vi "Wire Read Attributes.vi"(8 "error in (no error)":errorcluster, 9 "Controls":refnum<vi>[](array[refnum]), 10 "Cluster Refnum":refnum<vi>, 11 "VI in":refnum<vi>) -> (0 "error out":errorcluster, 3 "VI out":refnum<vi>)   [LabVIEW 2020, in "Message Maker.lvlib"]
uses:
  Message Maker.lvlib
  <vilib>/Utility/miscctls.llb/LVPositionTypeDef.ctl
  <vilib>/Utility/traverseref.llb/TRef TravTarget.ctl
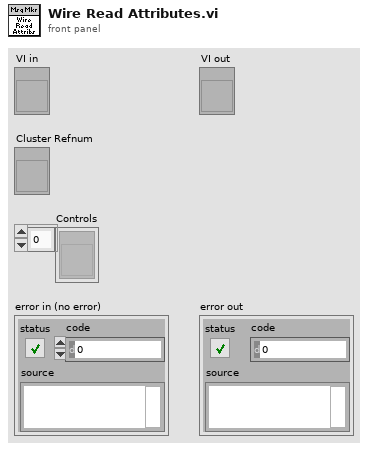
[diagram p1: front panel]
types:
  T1 = typedef "TRef TravTarget.ctl" = enum16{"FP", "BD", "Other"}
  T2 = typedef "LVPositionTypeDef.ctl" = cluster{"Left":i32, "Top":i32}
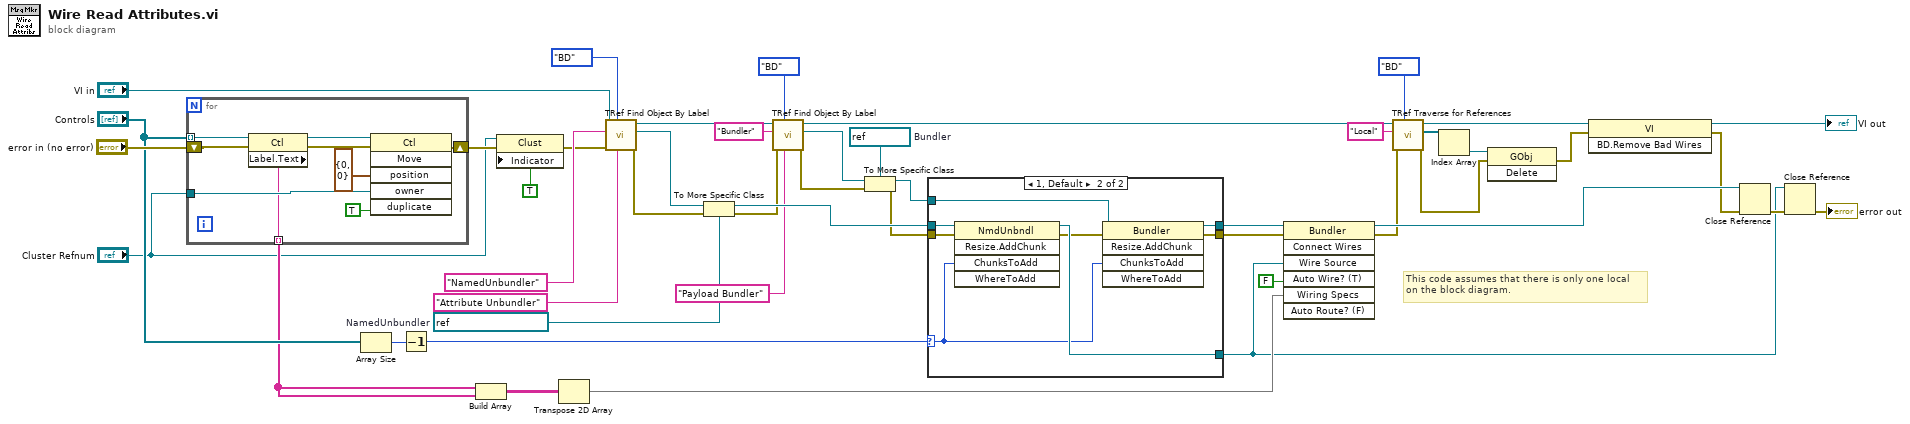
[diagram p0: block diagram]
diagram:
  w40 = refnum<vi> refnum  # Bundler
  w46 = refnum<vi> refnum  # NamedUnbundler
  # "This code assumes that there is only one local\non the block diagram."
  n1 = for {
    tunnel: "Cluster Refnum" -> [w55]
    tunnel: "Controls" -> [w54] mode=indexing
    shift-right: [w48] -> w4
    shift-left: "error in (no error)" -> [w52]
    tunnel: [w50] -> w35 mode=indexing
    n2 = property class="Ctl"(reference=w54, error in=w52) -> (reference out=w53:refnum<vi>, error out=w51:errorcluster, "Label.Text"=w50:string)
    n3 = invoke class="Ctl" method="Move"(reference=w53, error in=w51, "position"=T2 {"Left"=0, "Top"=0}, "owner"=w55, "duplicate"=TRUE ("Duplicate? (F)")) -> (error out=w48:errorcluster)  [unwired: 1 in, 5 out]
  }
  n4 = Array Size(array="Controls") -> (size(s)=w43:i32)
  n5 = Decrement(x=w43) -> (x-1=w19:i32)
  n6 = Build Array(w35, w35) -> (w33:string[][])
  n7 = property class="Clust"(reference="Cluster Refnum", error in=w4, "Indicator"=TRUE) -> (error out=w3:errorcluster)  [unwired: 1 out]
  n8 = Transpose 2D Array(2D array=w33) -> (transposed array=w32:string[][])
  n9 = call <vilib>:"TRef Find Object By Label.vi"("Label"="Attribute Unbundler", "Traverse Target"=TRef_TravTarget."BD", "error in (no error)"=w3, "Class Name"="NamedUnbundler", "VI Ref"="VI in") -> ("error out"=w5:errorcluster, "Found Obj Ref"=w14:refnum<vi>, "dup VI Ref"=w13:refnum<vi>)  [unwired: 3 in, 1 out]
  n10 = To More Specific Class(target class=w46, reference=w14, error in=w5) -> (specific class reference=w45:refnum<vi>, error out=w11:errorcluster)
  n11 = call <vilib>:"TRef Find Object By Label.vi"("Label"="Payload Bundler", "Traverse Target"=TRef_TravTarget."BD", "error in (no error)"=w11, "Class Name"="Bundler", "VI Ref"=w13) -> ("error out"=w6:errorcluster, "Found Obj Ref"=w9:refnum<vi>, "dup VI Ref"=w8:refnum<vi>)  [unwired: 3 in, 1 out]
  n12 = To More Specific Class(target class=w40, reference=w9, error in=w6) -> (specific class reference=w39:refnum<vi>, error out=w20:errorcluster)
  n13 = case shown="1, Default" w19 {
    selector: w19 -> [_ w60]
    tunnel: w45 -> [w59 w67]
    tunnel: w39 -> [w58 w66]
    tunnel: [w58 w65] -> w38
    tunnel: [w57 w64] -> w37
    tunnel: [w59 w63] -> w31
    tunnel: w20 -> [w57 w62]
    frame 0 {
    }
    frame 1, Default {
      n14 = invoke class="NmdUnbndl" method="Resize.AddChunk"(reference=w67, error in=w62, "ChunksToAdd"=w60) -> (reference out=w63:refnum<vi>, error out=w61:errorcluster)  [unwired: 2 in, 3 out]
      n15 = invoke class="Bundler" method="Resize.AddChunk"(reference=w66, error in=w61, "ChunksToAdd"=w60) -> (reference out=w65:refnum<vi>, error out=w64:errorcluster)  [unwired: 2 in, 3 out]
    }
  }
  n16 = invoke class="Bundler" method="Connect Wires"(reference=w38, error in=w37, "Wire Source"=w31, "Auto Wire? (T)"=FALSE, "Wiring Specs"=w32) -> (reference out=w36:refnum<vi>, error out=w28:errorcluster)  [unwired: 2 in, 5 out]
  n17 = call <vilib>:"TRef Traverse for References.vi"("Traverse Target"=TRef_TravTarget."BD", "error in (no error)"=w28, "Class Name"="Local", "VI Refnum"=w8) -> ("error out"=w24:errorcluster, "References"=w26:refnum<vi>[], "dup VI Refnum"=w29:refnum<vi>)  [unwired: 4 in, 1 out]
  n18 = Index Array(array=w26) -> (element=w25:refnum<vi>)  [unwired: 1 in]
  n19 = invoke class="GObj" method="Delete"(reference=w25, error in=w24) -> (error out=w22:errorcluster)  [unwired: 1 in, 2 out]
  n20 = invoke class="VI" method="BD.Remove Bad Wires"(reference=w29, error in=w22) -> (reference out=→"VI out":refnum<vi>, error out=w21:errorcluster)  [unwired: 1 in, 1 out]
  n21 = Close Reference(reference=w36, error in (no error)=w21) -> (error out=w42:errorcluster)
  n22 = Close Reference(reference=w31, error in (no error)=w42) -> (error out=→"error out":errorcluster)
